vi "multidev.vi"() -> ()   [LabVIEW 2011]
panel:
  out "Single Counts":i32[](array[numeric])
  out "Error Out":errorcluster
  out "Device Type":u16(ring) items=["No Device", "quTAG"]
  out "Serial Number":string
  out "Connected":bool
  out "Device ID":i32
  in  "Device Number":i32
  in  "stop":bool
  out "Device Count":i32
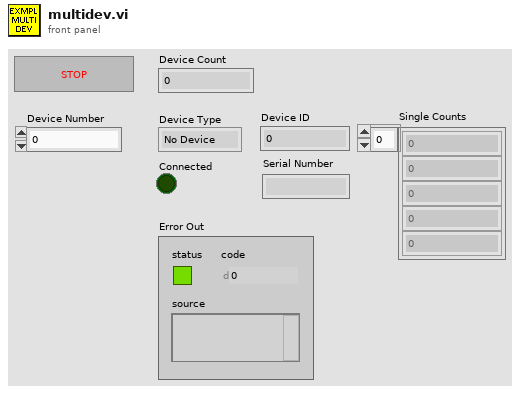
[diagram p1: front panel]
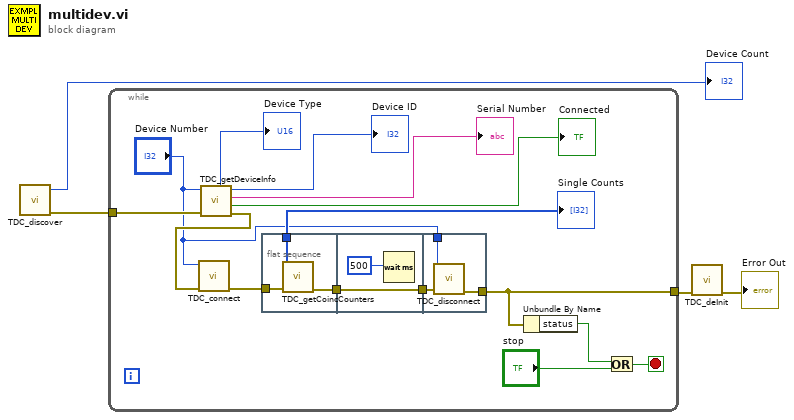
[diagram p0: block diagram]
diagram:
  n1 = call "TDC_discover.vi"() -> ("Error Out"=w3:errorcluster, "Device Count"=→"Device Count":i32)  [unwired: 10 in]
  n2 = while {
    tunnel: w3 -> [w17]
    tunnel: [w6] -> w1
    stop <- w18 stop-if-true
    n3 = call "TDC_getDeviceInfo.vi"("Error In"=w17, "Device Number"="Device Number") -> ("Error Out"=w12:errorcluster, "Connected"=→"Connected":bool, "Serial Number"=→"Serial Number":string, "Device ID"=→"Device ID":i32, "Device Type"=→"Device Type":u16)  [unwired: 5 in]
    n4 = call "TDC_connect.vi"("Error In"=w12, "Device Number"="Device Number") -> ("Error Out"=w11:errorcluster)  [unwired: 9 in]
    n5 = flat-sequence {
      tunnel: w11 -> [w22]
      tunnel: [w21] -> w9
      tunnel: [w20] -> w8
      tunnel: [w23] -> w10
      tunnel: w9 -> [w23]
      tunnel: w10 -> [w27]
      tunnel: "Device Number" -> [w26]
      tunnel: [w25] -> w6
      frame #0 {
        n6 = call "TDC_getCoincCounters.vi"("Error In"=w22) -> ("Error Out"=w21:errorcluster, "Single Counts"=w20:i32[])  [unwired: 4 in, 5 out]
      }
      frame #1 {
        n7 = Wait (ms)(milliseconds to wait=500) -> ()  [unwired: 1 out]
      }
      frame #2 {
        n8 = call "TDC_disconnect.vi"("Error In"=w27, "Device Number"=w26) -> ("Error Out"=w25:errorcluster)  [unwired: 9 in]
      }
    }
    n9 = Unbundle By Name(w6) -> ("status"=w5:bool)
    n10 = Or(x=w5, y="stop") -> (x .or. y?=w18:bool)
    "Single Counts" <- w8
  }
  n11 = call "TDC_deInit.vi"("Error In"=w1) -> ("Error Out"=→"Error Out":errorcluster)  [unwired: 10 in]
